vi "MPM_Connect.vi"(6 "GPIBBoard":i32, 8 "error in (no error)":errorcluster, 9 "Portnumber":i32, 10 "Address/ComPort":string, 11 "Communication":T1(ring)) -> (0 "error out":errorcluster, 3 "Reference out":refnum<k24>)   [LabVIEW 2017]
uses:
  C:/Users/Ssantec_Test/Documents/Instrument_DLL_Sample_Labview_20250826_Ver1.5.0_x64/DLL/InstrumentDLL.dll
  DLL/InstrumentDLL.dll
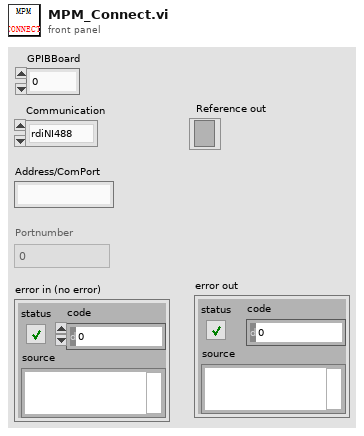
[diagram p1: front panel]
types:
  T1 = enum32{"rdiNI488", "rdiNIvisa", "rdikeysightvisa", "rdiLAN", "rdi232C"}
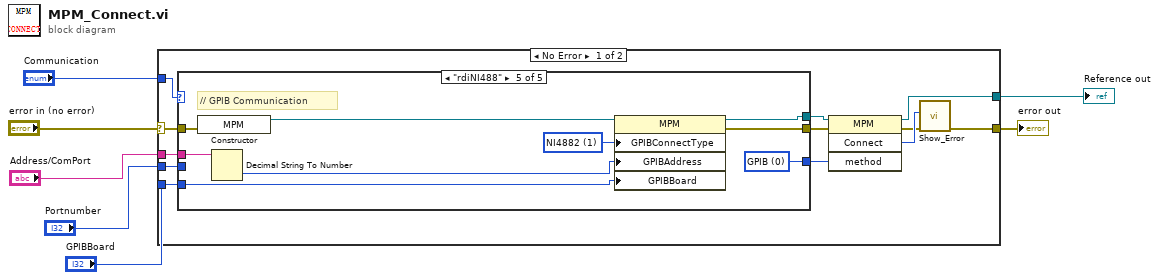
[diagram p0: block diagram]
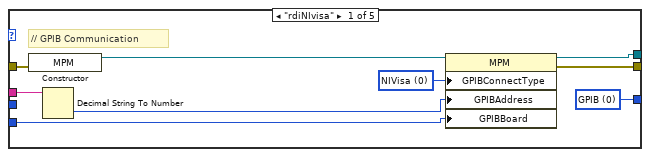
[diagram p2: hidden frame]
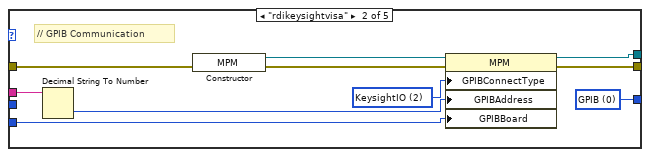
[diagram p3: hidden frame]
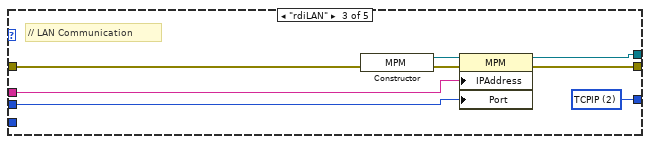
[diagram p4: hidden frame]
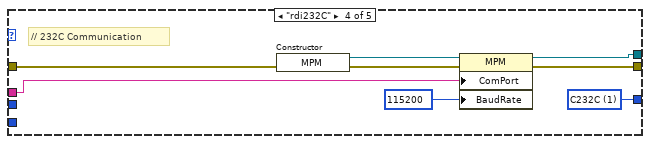
[diagram p5: hidden frame]
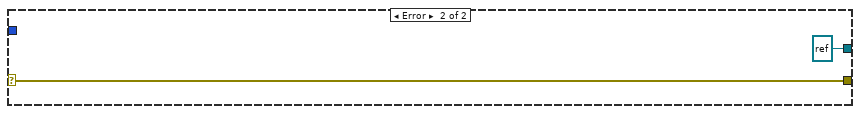
[diagram p6: hidden frame]
diagram:
  n1 = case shown="No Error" "error in (no error)" {
    selector: "error in (no error)" -> [w13 w64]
    tunnel: "Address/ComPort" -> [w19 _]
    tunnel: "Communication" -> [w18 _]
    tunnel: "Portnumber" -> [w17 _]
    tunnel: [w12 refnum<k24> refnum ("new reference")] -> w3
    tunnel: [w9 w64] -> w2
    tunnel: "GPIBBoard" -> [w8 _]
    frame No Error {
      n2 = case shown="\"rdiNI488\"" w18 {
        tunnel: w19 -> [w26 w36 w46 w52 w61]
        tunnel: w13 -> [w24 w34 w43 w50 w59]
        tunnel: w17 -> [_ _ w42 _ _]
        tunnel: [w23 w31 w41 w48 w58] -> w16
        tunnel: [w22 w32 w40 w47 w57] -> w15
        tunnel: [w21 w30 w39 w49 w56] -> w14
        tunnel: w8 -> [w20 w29 _ _ w55]
        frame "rdiNIvisa" {
          w21 = 0 items=["GPIB", "C232C", "TCPIP", "USB"] ("method")
          w28 = 0 items=["NIVisa", "NI4882", "KeysightIO"] ("GPIBConnectType")
          # "// GPIB Communication"
          n3 = constructor class="MPM"(error in=w24) -> (reference out=w25:refnum<k24>)  [unwired: 2 in, 2 out]
          n4 = Decimal String To Number(string=w26) -> (number=w27:i32)  [unwired: 2 in, 1 out]
          n5 = property on="属性节点" class="MPM"(reference=w25, "GPIBConnectType"=w28, "GPIBAddress"=w27, "GPIBBoard"=w20) -> (reference out=w23:refnum<k24>, error out=w22:errorcluster)  [unwired: 1 in]
        }
        frame "rdikeysightvisa" {
          w30 = 0 items=["GPIB", "C232C", "TCPIP", "USB"] ("method")
          w38 = 2 items=["NIVisa", "NI4882", "KeysightIO"] ("GPIBConnectType")
          # "// GPIB Communication"
          n6 = Decimal String To Number(string=w36) -> (number=w37:i32)  [unwired: 2 in, 1 out]
          n7 = constructor class="MPM"(error in=w34) -> (reference out=w35:refnum<k24>, error out=w33:errorcluster)  [unwired: 2 in, 1 out]
          n8 = property on="属性节点" class="MPM"(reference=w35, error in=w33, "GPIBConnectType"=w38, "GPIBAddress"=w37, "GPIBBoard"=w29) -> (reference out=w31:refnum<k24>, error out=w32:errorcluster)
        }
        frame "rdiLAN" {
          w39 = 2 items=["GPIB", "C232C", "TCPIP", "USB"] ("method")
          # "// LAN Communication"
          n9 = constructor class="MPM"(error in=w43) -> (reference out=w45:refnum<k24>, error out=w44:errorcluster)  [unwired: 2 in, 1 out]
          n10 = property on="属性节点" class="MPM"(reference=w45, error in=w44, "IPAddress"=w46, "Port"=w42) -> (reference out=w41:refnum<k24>, error out=w40:errorcluster)
        }
        frame "rdi232C" {
          w49 = 1 items=["GPIB", "C232C", "TCPIP", "USB"] ("method")
          # "// 232C Communication"
          n11 = constructor class="MPM"(error in=w50) -> (reference out=w54:refnum<k24>, error out=w51:errorcluster)  [unwired: 2 in, 1 out]
          n12 = property on="属性节点" class="MPM"(reference=w54, error in=w51, "ComPort"=w52, "BaudRate"=115200) -> (reference out=w48:refnum<k24>, error out=w47:errorcluster)
        }
        frame "rdiNI488" {
          w56 = 0 items=["GPIB", "C232C", "TCPIP", "USB"] ("method")
          w63 = 1 items=["NIVisa", "NI4882", "KeysightIO"] ("GPIBConnectType")
          # "// GPIB Communication"
          n13 = constructor class="MPM"(error in=w59) -> (reference out=w60:refnum<k24>)  [unwired: 2 in, 2 out]
          n14 = Decimal String To Number(string=w61) -> (number=w62:i32)  [unwired: 2 in, 1 out]
          n15 = property on="属性节点" class="MPM"(reference=w60, "GPIBConnectType"=w63, "GPIBAddress"=w62, "GPIBBoard"=w55) -> (reference out=w58:refnum<k24>, error out=w57:errorcluster)  [unwired: 1 in]
        }
      }
      n16 = invoke on="调用节点" class="MPM" method="Connect"(reference=w16, error in=w15, "method"=w14) -> (reference out=w12:refnum<k24>, error out=w10:errorcluster, "Connect"=w11:i32)  [unwired: 1 in, 1 out]
      n17 = call "Show_Error.vi"("error in (no error)"=w10, "Error"=w11) -> ("error out"=w9:errorcluster)  [unwired: 9 in]
    }
    frame Error {
    }
  }
  "error out" <- w2
  "Reference out" <- w3
